vi "Test Oxford ID and Read.vi"() -> ()   [LabVIEW 2016]
panel:
  out "Error Out":errorcluster
  out "read buffer":string
  in  "VISA resource name":refnum<visa-resource-name>="COM1"
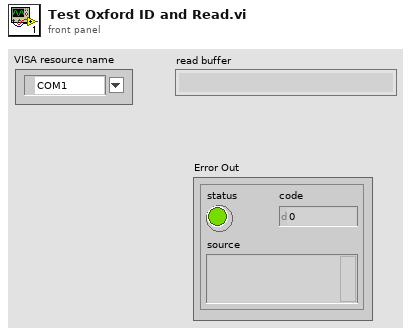
[diagram p1: front panel]
types:
  T1 = typedef "Device type.ctl" = enum16{"NONE", "Neocera 21", "LakeShore 335", "LakeShore 336", "LakeShore 340", "LkShr 340 chA&B", "LakeShore 370", "SRS 850", "SRS 830", "LR 700", "EG&G 5302", "EG&G 7260", "EG&G 7280", "AH 2500", "Keithley meter", "Keithley electrometer", "Keithley 182", "HP 5385", "HP 53181", "HP 53132", "ITC503", "IPS120", "Oxford Mercury IPS", "Oxford PS", "Test", "DC Facility Magnet", "Cryomagnetics PS", "Keithley 2400", "Keithley current source", "Cryo-Con 22C", "HP87NN", "HP4395A", "Agilent 34410A"}
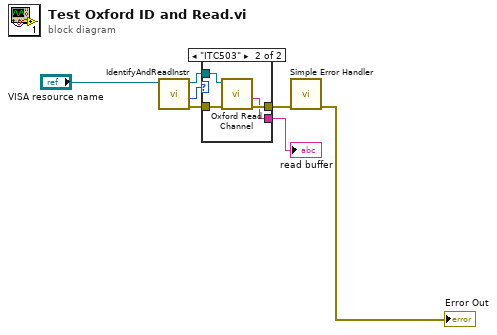
[diagram p0: block diagram]
diagram:
  n1 = call "IdentifyAndReadInstr.vi"("VISA Resource Name"="VISA resource name") -> ("error out"=w4:errorcluster, "Instrument"=w6:T1, "VISA Resource Name Out"=w5:refnum<visa-resource-name>)  [unwired: 7 in, 1 out]
  n2 = case shown="\"ITC503\"" w6 {
    tunnel: w5 -> [_ w12]
    tunnel: w4 -> [w8 w11]
    tunnel: [w8 w10] -> w3
    tunnel: [_ w9] -> w2
    frame "NONE", Default {
    }
    frame "ITC503" {
      n3 = call "Oxford Read Channel.vi"("error in (no error)"=w11, "VISA resource name"=w12) -> ("error out"=w10:errorcluster, "read buffer"=w9:string)  [unwired: 6 in, 2 out]
    }
  }
  "read buffer" <- w2
  n4 = call <vilib>:"Simple Error Handler.vi"("error in (no error)"=w3) -> ("error out"=→"Error Out":errorcluster)  [unwired: 4 in, 4 out]
